vi "WriteWaveformAndMap.vi"(8 "error in (no error)":errorcluster, 10 "data":T1, 11 "config":variant) -> (0 "error out":errorcluster, 1 "first block":bool, 2 "block number":u32)   [LabVIEW 2017, in "DVRBuffer.lvlib"]
uses:
  <vilib>/addons/InsightCM/Devices/Shared/Common/DVRBuffer/DVRBuffer.lvlib
  <vilib>/addons/InsightCM/Devices/Shared/Common/DataFlow/controls/Data.ctl
  <vilib>/addons/InsightCM/Utilities/DataAccessors/controls/wfmSGL_DVR.ctl
  <vilib>/addons/PointValueMap/controls/PointMap.ctl
  <vilib>/addons/InsightCM/Devices/Shared/Common/DataFlow/controls/Type.ctl
  <vilib>/addons/InsightCM/Devices/Shared/Common/DVRBuffer/controls/InternalDataType_waveformmap.ctl
  <vilib>/addons/InsightCM/Devices/Shared/Common/DVRBuffer/controls/DVRElement.ctl
  <vilib>/addons/InsightCM/Devices/Shared/Common/DataAccumulator/controls/config.ctl
  <vilib>/addons/InsightCM/Devices/Shared/Common/DeviceHealth/controls/deviceHealthTag.ctl
  <vilib>/addons/InsightCM/Devices/Shared/Common/DeviceHealth/controls/SystemHealthTagEnum.ctl
  <vilib>/addons/InsightCM/MessageBus/Base/controls/Tag.ctl
  <vilib>/addons/InsightCM/MessageBus/Base/controls/KeyValuePair.ctl
  <vilib>/addons/PointValueMap/subVIs/Point_Read_i32.vi
  <vilib>/addons/PointValueMap/PointValueMap.lvlib
  <vilib>/addons/InsightCM/Devices/Shared/Common/DataAccumulator/DataAccumulator.lvlib
  <vilib>/addons/InsightCM/Devices/Shared/Common/DeviceHealth/DeviceHealth.lvlib
  <vilib>/addons/InsightCM/Devices/Shared/Common/DataFlow/DataFlow.lvlib
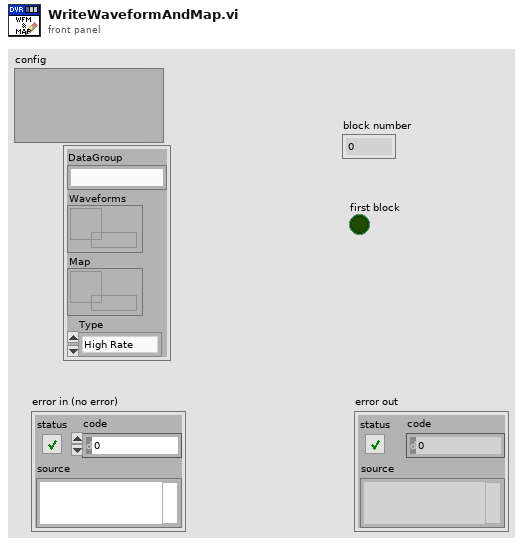
[diagram p1: front panel]
types:
  T1 = typedef "DataFlow.lvlib/Data.ctl" = cluster{"DataGroup":string, "Waveforms":T2, "Map":T3, "Type":T4}
  T2 = typedef "wfmSGL_DVR.ctl" = refnum<data-value>
  T3 = typedef "PointValueMap.lvlib/PointMap.ctl" = refnum<data-value>
  T4 = typedef "DataFlow.lvlib/Type.ctl" = enum16{"High Rate", "Low Rate", "Burst Mode"}
  T5 = typedef "DataAccumulator.lvlib/config.ctl" = cluster{"Group":string, "BlockComplete":bool, "Ok To Start":bool, "Speed Ref Chan":string, "Current OpState":string, "MaxLowRateCPU(%)":dbl, "MaxLowRateMem(%)":dbl, "LowRateCount":i32, "LowRateCountTag":T6}
  T6 = typedef "DeviceHealth.lvlib/deviceHealthTag.ctl" = cluster{"SystemTags":T7, "TagId":string, "Tag":T8}
  T7 = typedef "DeviceHealth.lvlib/SystemHealthTagEnum.ctl" = enum16{"CPU Utilization", "Memory Utilization", "Disk Utilization", "Total Physical Memory", "Primary Disk Free", "Chassis Temperature", "LowRateCount"}
  T8 = typedef "Tag.ctl" = cluster{"Id":string, "Path":string, "Name":string, "Datatype":string, "Props":T9[], "Keywords":string[]}
  T9 = typedef "KeyValuePair.ctl" = cluster{"Key":string, "Value":string}
  T10 = typedef "DVRBuffer.lvlib/DVRElement.ctl" = cluster{"location":u32, "DVR":u32, "points":i32, "dt":dbl, "PulsePositions":dbl[], "Pulses Per Rev":dbl}
  T11 = typedef "DVRBuffer.lvlib/InternalDataType_waveformmap.ctl" = cluster{"waveforms":waveform(sgl)[], "map":T3}
  T12 = typedef "AnalysisHelper.lvlib/PulsePositions.ctl" = cluster{"Name":string, "Pulse Position Data":dbl[], "Pulses Per Rev":i32}
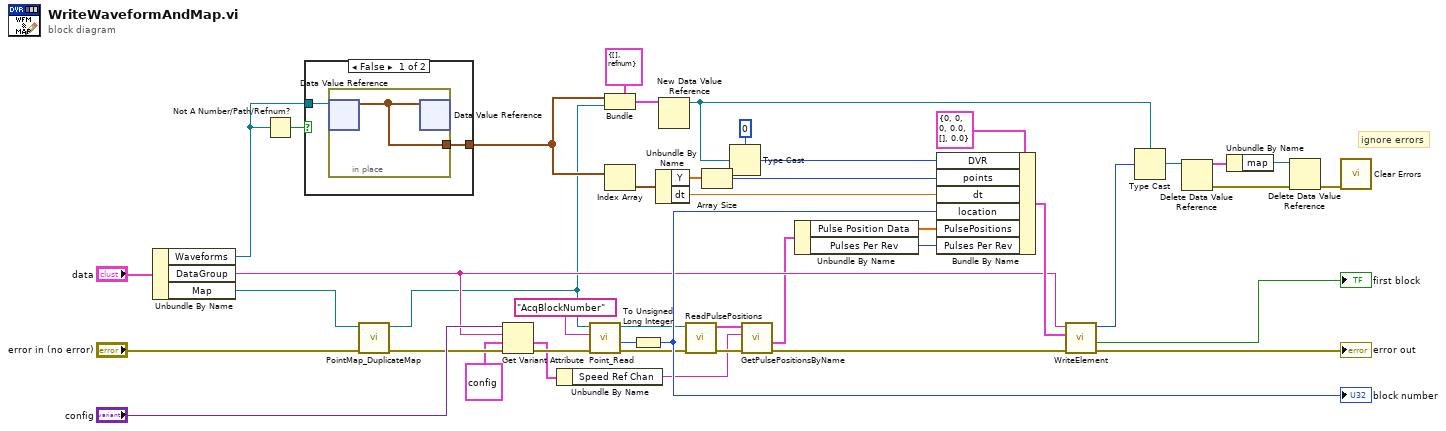
[diagram p0: block diagram]
diagram:
  # "ignore errors"
  n1 = Unbundle By Name("data") -> ("Waveforms"=w2:T2, "DataGroup"=w17:string, "Map"=w3:T3)
  n2 = Not A Number/Path/Refnum?(number/path/refnum=w2) -> (NaN/Path/Refnum?=w7:bool)
  n3 = case shown="False" w7 {
    tunnel: w2 -> [w46 _]
    tunnel: [w45 _] -> w8
    frame False {
      n4 = in-place {
        in-place-border: [w47] -> w45
        n5 = in-place-dvr #1(w46) -> (w47:waveform(sgl)[])  [unwired: 1 out]
        n6 = in-place-dvr #1(w47) -> ()  [unwired: 2 out]
      }
    }
    frame True {
    }
  }
  n7 = call <vilib>:"PointMap_DuplicateMap.vi"("error in (no error)"="error in (no error)", "map in"=w3) -> ("error out"=w5:errorcluster, "duplicate map"=w4:T3)  [unwired: 8 in]
  n8 = Get Variant Attribute(Variant="config", name=w17, default value (empty Variant)=T5 {"Group"="", "BlockComplete"=FALSE, "Ok To Start"=FALSE, "Speed Ref Chan"="", "Current OpState"="", "MaxLowRateCPU(%)"=0.0, "MaxLowRateMem(%)"=0.0, "LowRateCount"=0, "LowRateCountTag"={"SystemTags"=enum."CPU Utilization", "TagId"="", "Tag"={"Id"="", "Path"="", "Name"="", "Datatype"="", "Props"=[], "Keywords"=[]}}} ("Config"), error in=w5) -> (value=w16:T5, error out=w19:errorcluster)  [unwired: 2 out]
  n9 = Unbundle By Name(w16) -> ("Speed Ref Chan"=w12:string)
  n10 = call-poly <vilib>:"Point_Read.vi"("Error In"=w19, "Tag"="AcqBlockNumber", "Map"=w4) -> ("Error Out"=w20:errorcluster, "Value"=w30:i32, "Map Out"=w21:T3)  [unwired: 3 in, 3 out]
  n11 = Bundle(cluster=T11 {"waveforms"=[], "map"=refnum} ("output cluster"), "waveforms"=w8, "map"=w4) -> (w39:T11)
  n12 = Index Array(array=w8) -> (element=w27:waveform(sgl))  [unwired: 1 in]
  n13 = To Unsigned Long Integer(number=w30) -> (unsigned 32bit integer=w22:u32)
  "block number" <- w22
  n14 = Unbundle By Name(w27) -> ("Y"=w26:sgl[], "dt"=w24:dbl)
  n15 = New Data Value Reference(data value=w39) -> (data value reference=w42:refnum<data-value>)  [unwired: 1 in, 1 out]
  n16 = call <vilib>:"ReadPulsePositions.vi"("error in (no error)"=w20, "Map"=w21) -> ("error out"=w14:errorcluster, "pulse positions array"=w15:T12[])  [unwired: 7 in, 1 out]
  n17 = Array Size(array=w26) -> (size(s)=w25:i32)
  n18 = Type Cast(type=u32 0, x=w42) -> (*(type *) &x=w28:u32)
  n19 = call <vilib>:"GetPulsePositionsByName.vi"("error in (no error)"=w14, "Channel Name"=w12, "Pulse Positions Array"=w15) -> ("error out"=w13:errorcluster, "Pulse Positions"=w11:T12)  [unwired: 5 in, 2 out]
  n20 = Unbundle By Name(w11) -> ("Pulse Position Data"=w10:dbl[], "Pulses Per Rev"=w9:i32)
  n21 = Bundle By Name(cluster=T10 {"location"=0, "DVR"=0, "points"=0, "dt"=0.0, "PulsePositions"=[], "Pulses Per Rev"=0.0} ("DVR element"), "DVR"=w28, "points"=w25, "dt"=w24, "location"=w22, "PulsePositions"=w10, "Pulses Per Rev"=w9) -> (w29:T10)
  n22 = call <vilib>:"WriteElement.vi"("error in (no error)"=w13, "dvr element"=w29, "name"=w17) -> ("error out"=→"error out":errorcluster, "initialize"=→"first block":bool, "replaced dvr"=w43:u32)  [unwired: 6 in]
  n23 = Type Cast(type=w42, x=w43) -> (*(type *) &x=w41:refnum<data-value>)
  n24 = Delete Data Value Reference(data value reference=w41) -> (data value=w38:T11, error out=w36:errorcluster)  [unwired: 1 in]
  n25 = Unbundle By Name(w38) -> ("map"=w37:T3)
  n26 = Delete Data Value Reference(data value reference=w37, error in=w36) -> (error out=w35:errorcluster)  [unwired: 1 out]
  n27 = call <vilib>:"Clear Errors.vi"("error in (no error)"=w35) -> ()  [unwired: 5 in, 2 out]
